vi "lsl protocol version.vi"(8 "error in (no error)":errorcluster) -> (0 "error out":errorcluster, 3 "function return":i32)   [LabVIEW 2018, in "liblsl-LabVIEW.lvlib"]
doc: "extern LIBLSL_C_API int32_t lsl_protocol_version();"
uses:
  <userlib>/liblsl-LabVIEW/liblsl-LabVIEW.lvlib
  <userlib>/liblsl-LabVIEW/liblsl64.dll
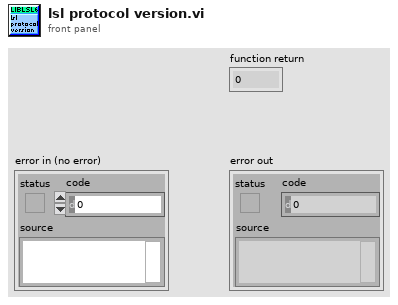
[diagram p1: front panel]
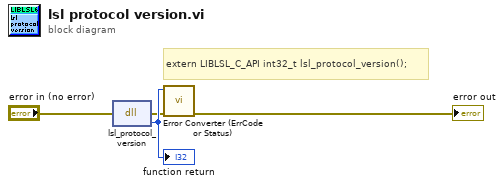
[diagram p0: block diagram]
diagram:
  # "extern LIBLSL_C_API int32_t lsl_protocol_version();"
  n1 = dll-call lib="C:/Program Files/National Instruments/LabVIEW 2018/user.lib/liblsl-LabVIEW/liblsl64.*" fn="lsl_protocol_version"(error in="error in (no error)") -> (error out=w2:errorcluster, w4:i32)  [unwired: 2 in, 1 out]
  "function return" <- w4
  n2 = call <userlib>:"Error Converter (ErrCode or Status).vi"("error in (no error)"=w2, "error code"=w4) -> ("error out"=→"error out":errorcluster)  [unwired: 9 in]
